vi "Deadband Calibrations.vi"() -> ()   [LabVIEW 2016]
panel:
  out "Robot Twist Multiplier":dbl
  in  "Deadband Calibrations File Location":path=path "C:/ni-rt/startup/DeadbandCalibrations.txt"
  out "Robot Forward-Back Deadband (throttle)":dbl
  out "Robot Twist Deadband (throttle)":dbl
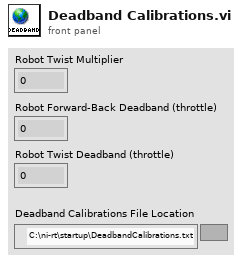
[diagram p1: front panel]
diagram:
